vi "AlliGator skippable_Delete Existing ROIs Dialog Window.vi"(8 "Error In":errorcluster) -> (0 "Error Out":errorcluster, 3 "Delete":bool)   [LabVIEW 2021, in "AlliGator GUI.lvlib"]
doc: "Asks the user whether the existing ROIs should be kept or deleted before loading the new ones.\n\nThis dialog is skippable by clicking on a checkbox, but can be re-activated by going to Settings?Miscellaneous."
uses:
  <vilib>/Utility/miscctls.llb/LVKeyNavTypeDef.ctl
  <vilib>/Utility/error.llb/Error Cluster From Error Code.vi
  <vilib>/ErrorRing/Error Ring.xnode
  GUI/AlliGator GUI.lvlib
panel:
  in  "Do not show this dialog again":bool
  in  "Return Key association":enum32{"Delete", "Add"}(radio)
  in  "Add":bool
  in  "Delete":bool
  out "Displayed Message":string="Delete existing ROIs, or keep them and add the new ones?"
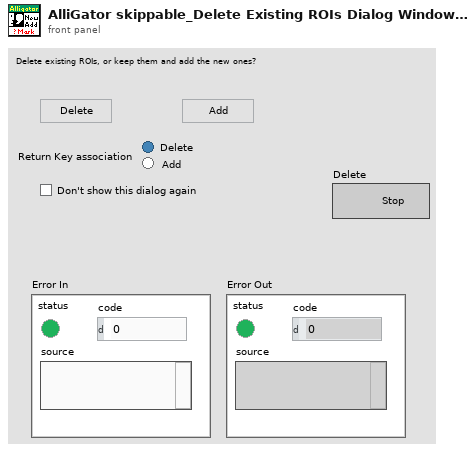
[diagram p1: front panel]
types:
  T1 = typedef "LVKeyNavTypeDef.ctl" = cluster{"Control":bool, "Shift":bool, "Key":string}
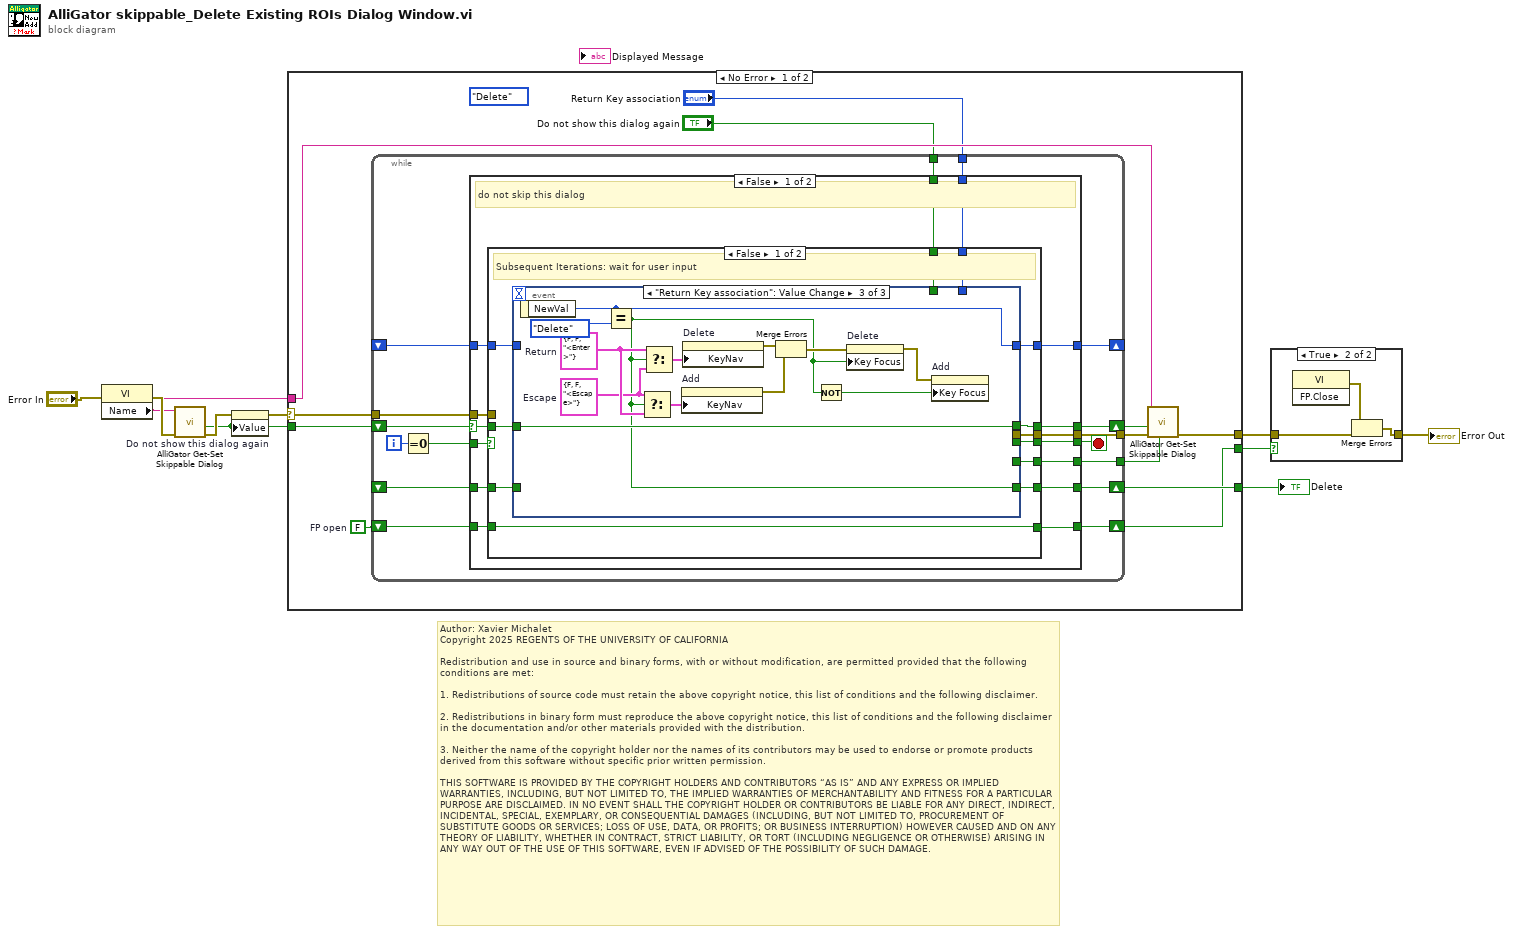
[diagram p0: block diagram]
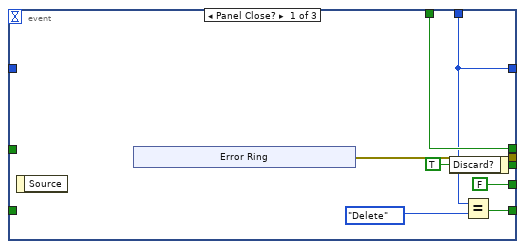
[diagram p3: hidden frame]
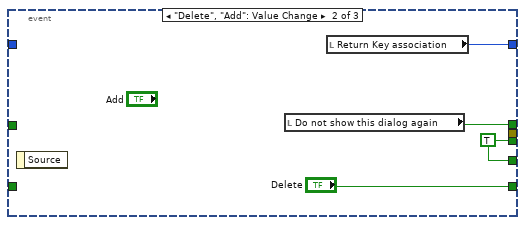
[diagram p4: hidden frame]
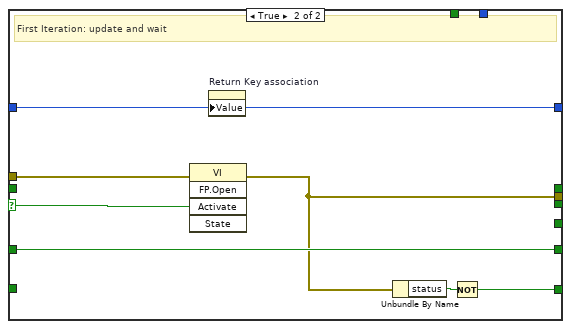
[diagram p5: hidden frame]
diagram:
  # "Author: Xavier Michalet\nCopyright 2025 REGENTS OF THE UNIVERSITY OF CALIFORNIA\n\nRedistribution and use in source and binary forms, with or without modification, are permitted provided that the following conditions are met:\n\n1. Redistributions of source code must retain the above copyright notice, this list of conditions and the following disclaimer.\n\n2. Redistributions in binary form must reproduce the above copyright notice, this list of conditions and the following disclaimer in the documentation and/or other materials provided with the distribution.\n\n3. Neither the name of the copyright holder nor the names of its contributors may be used to endorse or promote products derived from this software without specific prior written permission.\n\nTHIS SOFTWARE IS PROVIDED BY THE COPYRIGHT HOLDERS AND CONTRIBUTORS “AS IS” AND ANY EXPRESS OR IMPLIED WARRANTIES, INCLUDING, BUT NOT LIMITED TO, THE IMPLIED WARRANTIES OF MERCHANTABILITY AND FITNESS FOR A PARTICULAR PURPOSE ARE DISCLAIMED. IN NO EVENT SHALL THE COPYRIGHT HOLDER OR CONTRIBUTORS BE LIABLE FOR ANY DIRECT, INDIRECT, INCIDENTAL, SPECIAL, EXEMPLARY, OR CONSEQUENTIAL DAMAGES (INCLUDING, BUT NOT LIMITED TO, PROCUREMENT OF SUBSTITUTE GOODS OR SERVICES; LOSS OF USE, DATA, OR PROFITS; OR BUSINESS INTERRUPTION) HOWEVER CAUSED AND ON ANY THEORY OF LIABILITY, WHETHER IN CONTRACT, STRICT LIABILITY, OR TORT (INCLUDING NEGLIGENCE OR OTHERWISE) ARISING IN ANY WAY OUT OF THE USE OF THIS SOFTWARE, EVEN IF ADVISED OF THE POSSIBILITY OF SUCH DAMAGE."
  n1 = property class="VI"(error in="Error In") -> (error out=w9:errorcluster, "Name"=w7:string)  [unwired: 1 in, 1 out]
  n2 = call "AlliGator Get-Set Skippable Dialog.vi"("Error In"=w9, "Dialog Window VI Name"=w7) -> ("Error Out"=w6:errorcluster, "Is skipped (out)"=w4:bool)  [unwired: 8 in]
  n3 = property on="Do not show this dialog again" class="Bool (strict)"(error in=w6, "Value"=w4) -> (error out=w5:errorcluster)  [unwired: 1 in, 1 out]
  n4 = case shown="No Error" w5 {
    selector: w5 -> [w12 w106]
    tunnel: [w22 _] -> w10
    tunnel: [w18 w106] -> w8
    tunnel: w4 -> [w21 _]
    tunnel: w7 -> [w20 _]
    tunnel: [w13 _] -> w3
    frame No Error {
      (unwired) enum32{"Delete", "Add"}."Delete" ("Return Key association")
      w14 = FALSE  # FP open
      n5 = while {
        shift-right: [w35] -> _
        shift-left: _ -> [w36]
        shift-right: [w37] -> w22
        shift-left: _ -> [w34]
        shift-right: [w33] -> w19
        shift-left: w21 -> [w27]
        tunnel: "Do not show this dialog again" -> [w32]
        tunnel: [w31] -> w16
        tunnel: "Return Key association" -> [w30]
        shift-right: [w25] -> w13
        shift-left: w14 -> [w26]
        tunnel: w12 -> [w24]
        tunnel: [w23] -> w11
        i -> [w29]
        stop <- w38 stop-if-true
        n6 = Equal To 0?(x=w29) -> (x = 0?=w28:bool)
        n7 = case shown="False" w27 {
          selector: w27 -> [w43 w104]
          tunnel: [w53 w104] -> w38
          tunnel: [w52 w103] -> w37
          tunnel: w36 -> [w51 w105]
          tunnel: [w50 w105] -> w35
          tunnel: w34 -> [w49 w103]
          tunnel: [w48 w104] -> w33
          tunnel: w32 -> [w47 _]
          tunnel: [w46 w104] -> w31
          tunnel: w30 -> [w45 _]
          tunnel: w28 -> [w44 _]
          tunnel: w26 -> [w42 w102]
          tunnel: [w39 w102] -> w25
          tunnel: w24 -> [w41 w101]
          tunnel: [w40 w101] -> w23
          frame False {
            # "do not skip this dialog"
            n8 = case shown="False" w44 {
              selector: w44 -> [_ w100]
              tunnel: [w65 _] -> w53
              tunnel: [w64 w98] -> w52
              tunnel: [w63 w99] -> w50
              tunnel: w51 -> [w62 w99]
              tunnel: w49 -> [w57 w98]
              tunnel: [w61 _] -> w48
              tunnel: w47 -> [w60 _]
              tunnel: w43 -> [w56 _]
              tunnel: [w58 _] -> w46
              tunnel: w45 -> [w59 _]
              tunnel: w42 -> [w55 _]
              tunnel: w41 -> [_ w96]
              tunnel: [w54 w95] -> w40
              tunnel: [w55 w94] -> w39
              frame False {
                # "Subsequent Iterations: wait for user input"
                n9 = event shown="[2] \"Return Key association\": Value Change" {
                  selector: _ -> [_ _ _]
                  dyn-events: _ -> [_ _ _]
                  timeout: _ -> [_ _ _]
                  tunnel: [w72 w78 _] -> w65
                  tunnel: [w68 "Delete" w82] -> w64
                  tunnel: [w69 w77 w84] -> w63
                  tunnel: w62 -> [_ _ _]
                  tunnel: [w71 w79 w83] -> w61
                  tunnel: w60 -> [w71 _ _]
                  tunnel: w59 -> [w69 _ _]
                  tunnel: [FALSE ("Discard?") w78 _] -> w58
                  tunnel: w57 -> [_ _ _]
                  tunnel: w56 -> [_ _ w83]
                  tunnel: [w67 _ _] -> w54
                  event Panel Close? {
                    w72 = TRUE ("Discard?")
                    n10 = event-data() -> ()  [unwired: 1 in, 1 out]
                    n11 = xnode "Error Ring"() -> ("error out"=w67:errorcluster)
                    n12 = event-data("Discard?"=w72) -> ()  [unwired: 1 in, 1 out]
                    n13 = Equal?(x=w69, y=enum32{"Delete", "Add"}."Delete" ("Return Key association")) -> (x = y?=w68:bool)
                  }
                  event "Delete", "Add": Value Change {
                    w78 = TRUE ("Discard?")
                    n14 = event-data() -> ()  [unwired: 1 in, 1 out]
                    n15 = local read "Do not show this dialog again"() -> (w79:bool)
                    n16 = local read "Return Key association"() -> (w77:enum32{"Delete", "Add"})
                  }
                  event "Return Key association": Value Change {
                    w90 = T1 {"Control"=FALSE, "Shift"=FALSE, "Key"="<Escape>"}  # Escape
                    w91 = T1 {"Control"=FALSE, "Shift"=FALSE, "Key"="<Enter>"}  # Return
                    n17 = event-data() -> ("NewVal"=w84:enum32{"Delete", "Add"})  [unwired: 1 in]
                    n18 = Equal?(x=w84, y=enum32{"Delete", "Add"}."Delete" ("Return Key association")) -> (x = y?=w82:bool)
                    n19 = Select(t=w90, s=w82, f=w91) -> (s? t:f=w93:T1)
                    n20 = Select(t=w91, s=w82, f=w90) -> (s? t:f=w92:T1)
                    n21 = property on="Add" class="Bool"("KeyNav"=w93) -> (error out=w87:errorcluster)  [unwired: 2 in, 1 out]
                    n22 = property on="Delete" class="Bool"("KeyNav"=w92) -> (error out=w88:errorcluster)  [unwired: 2 in, 1 out]
                    n23 = Merge Errors(w88, w87) -> (w86:errorcluster)
                    n24 = Not(x=w82) -> (.not. x?=w89:bool)
                    n25 = property on="Delete" class="Bool"(error in=w86, "Key Focus"=w82) -> (error out=w85:errorcluster)  [unwired: 1 in, 1 out]
                    n26 = property on="Add" class="Bool"(error in=w85, "Key Focus"=w89) -> ()  [unwired: 1 in, 2 out]
                  }
                }
              }
              frame True {
                # "First Iteration: update and wait"
                n27 = invoke class="VI" method="FP.Open"(error in=w96, "Activate"=w100) -> (error out=w95:errorcluster)  [unwired: 3 in, 4 out]
                n28 = property on="Return Key association" class="RadioBtnsControl (strict)"("Value"=w99) -> ()  [unwired: 2 in, 2 out]
                n29 = Unbundle By Name(w95) -> ("status"=w97:bool)
                n30 = Not(x=w97) -> (.not. x?=w94:bool)
              }
            }
          }
          frame True {
            # "skip this dialog if first call only"
          }
        }
      }
      n31 = call "AlliGator Get-Set Skippable Dialog.vi"("Set/Get (F)"=w16, "Error In"=w11, "Is skipped (in)"=w19, "Dialog Window VI Name"=w20) -> ("Error Out"=w18:errorcluster)  [unwired: 6 in, 1 out]
    }
    frame Error {
    }
  }
  "Delete" <- w10
  n32 = case shown="True" w3 {
    tunnel: w8 -> [w107 w108]
    tunnel: [w107 w109] -> w1
    frame False {
    }
    frame True {
      n33 = invoke class="VI" method="FP.Close"() -> (error out=w110:errorcluster)  [unwired: 3 in, 2 out]
      n34 = Merge Errors(w110, w108) -> (w109:errorcluster)
    }
  }
  "Error Out" <- w1
